vi "Get Symbol.vi"(8 "error in (no error)":errorcluster, 11 "Symbol in":refnum<class "Symbol.lvclass">) -> (0 "error out":errorcluster, 2 "Symbol":string, 3 "Symbol out":refnum<class "Symbol.lvclass">)   [LabVIEW 2020, in "Symbol.lvclass"]
uses:
  Symbol.lvclass
  Symbol.lvclass/Symbol.ctl
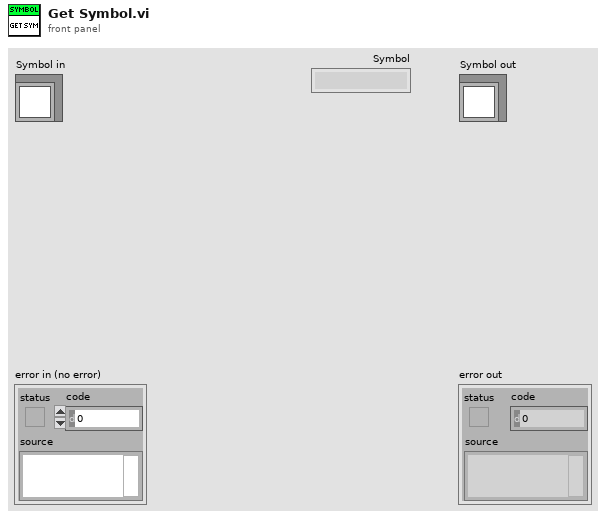
[diagram p1: front panel]
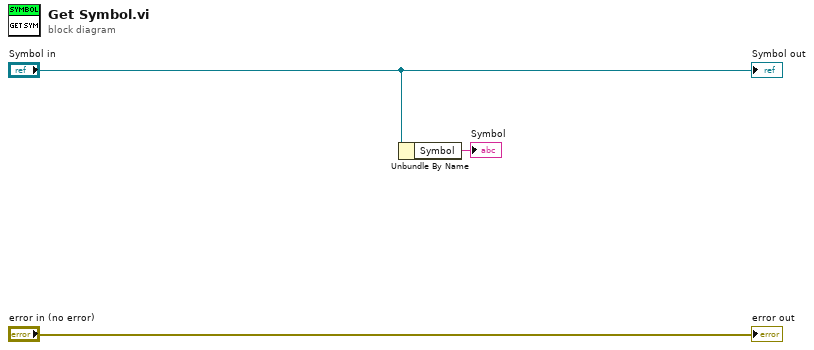
[diagram p0: block diagram]
diagram:
  n1 = Unbundle By Name("Symbol in") -> ("Symbol"=→"Symbol":string)
  "error out" <- "error in (no error)"
  "Symbol out" <- "Symbol in"
